vi "Initialize.vi"(8 "error in":errorcluster, 11 "Plugin in":refnum<class "Power Spectrum Density.lvclass">) -> (0 "error out":errorcluster, 3 "Plugin out":refnum<class "Power Spectrum Density.lvclass">)   [LabVIEW 2023, in "Power Spectrum Density.lvlib" / "Power Spectrum Density.lvclass"]
uses:
  Power Spectrum Density.lvclass
  C:/Program Files/National Instruments/LabVIEW 2023/vi.lib/FlexLogger/SDK/PluginSDK.lvlibp/PEFClasses/SDK/Plugin/Plugin.lvclass
  Power Spectrum Density Global.vi
  <vilib>/FlexLogger/SDK/PluginSDK.lvlibp/PEFClasses/SDK/Plugin/ParameterAccess/Write Single Channel.vi
  <vilib>/FlexLogger/SDK/PluginSDK.lvlibp/PEFClasses/SDK/Plugin/ParameterAccess/Write Enum.vi
  <vilib>/FlexLogger/SDK/PluginSDK.lvlibp/PEFClasses/SDK/Plugin/ParameterAccess/Write Boolean.vi
  <vilib>/FlexLogger/SDK/PluginSDK.lvlibp/PEFClasses/SDK/Plugin/ParameterAccess/Write I32.vi
  <vilib>/FlexLogger/SDK/PluginSDK.lvlibp/PEFClasses/SDK/Plugin/ParameterAccess/Write DBL.vi
  <vilib>/FlexLogger/SDK/PluginSDK.lvlibp/PEFClasses/SDK/Plugin/ParameterAccess/Write Command.vi
  <vilib>/FlexLogger/SDK/PluginSDK.lvlibp/PEFClasses/SDK/Plugin/Plugin.lvclass
  C:/Program Files/National Instruments/LabVIEW 2023/vi.lib/FlexLogger/SDK/PluginSDK.lvlibp/PEFClasses/SDK/Processing Element/Processing Element.lvclass
  C:/Users/Administrator/Documents/LabVIEW Projects/FlexLogger IO Plug-ins/Power Spectrum Density/Power Spectrum Density.lvclass
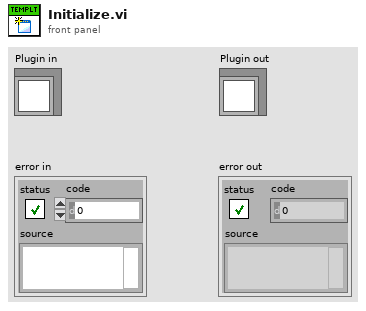
[diagram p1: front panel]
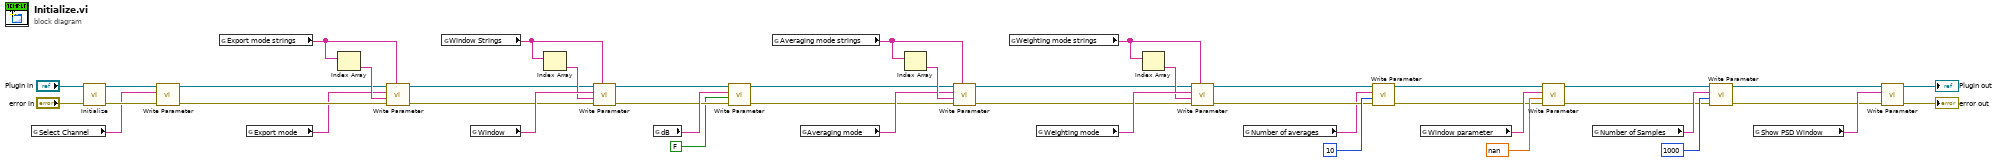
[diagram p0: block diagram]
diagram:
  n1 = global read "Power Spectrum Density Global.vi" "Select Channel"() -> (w38:string)
  n2 = call-parent "Initialize.vi"("error in (no error)"="error in", "Plugin in"="Plugin in") -> ("error out"=w39:errorcluster, "Plugin out"=w40:refnum<class "Power Spectrum Density.lvclass">)  [unwired: 8 in]
  n3 = call-poly <vilib>:"Write Parameter.vi"("error in (no error)"=w39, "Name (Unique Channel Identifier)"=w38, "Plugin in"=w40) -> ("error out"=w41:errorcluster, "Plugin out"=w42:refnum<class "Power Spectrum Density.lvclass">)  [unwired: 7 in]
  n4 = global read "Power Spectrum Density Global.vi" "Export mode strings"() -> (w37:string[])
  n5 = global read "Power Spectrum Density Global.vi" "Export mode"() -> (w36:string)
  n6 = Index Array(array=w37) -> (element=w43:string)  [unwired: 1 in]
  n7 = call-poly <vilib>:"Write Parameter.vi"("Possible Values"=w37, "error in (no error)"=w41, "Current Value"=w43, "Name"=w36, "Plugin in"=w42) -> ("error out"=w29:errorcluster, "Plugin out"=w30:refnum<class "Power Spectrum Density.lvclass">)  [unwired: 5 in]
  n8 = global read "Power Spectrum Density Global.vi" "Window Strings"() -> (w32:string[])
  n9 = global read "Power Spectrum Density Global.vi" "Window"() -> (w33:string)
  n10 = Index Array(array=w32) -> (element=w31:string)  [unwired: 1 in]
  n11 = call-poly <vilib>:"Write Parameter.vi"("Possible Values"=w32, "error in (no error)"=w29, "Current Value"=w31, "Name"=w33, "Plugin in"=w30) -> ("error out"=w26:errorcluster, "Plugin out"=w27:refnum<class "Power Spectrum Density.lvclass">)  [unwired: 5 in]
  n12 = global read "Power Spectrum Density Global.vi" "dB"() -> (w28:string)
  n13 = call-poly <vilib>:"Write Parameter.vi"("error in (no error)"=w26, "Value"=FALSE, "Name"=w28, "Plugin in"=w27) -> ("error out"=w17:errorcluster, "Plugin out"=w18:refnum<class "Power Spectrum Density.lvclass">)  [unwired: 6 in]
  n14 = global read "Power Spectrum Density Global.vi" "Averaging mode strings"() -> (w23:string[])
  n15 = global read "Power Spectrum Density Global.vi" "Averaging mode"() -> (w22:string)
  n16 = Index Array(array=w23) -> (element=w24:string)  [unwired: 1 in]
  n17 = call-poly <vilib>:"Write Parameter.vi"("Possible Values"=w23, "error in (no error)"=w17, "Current Value"=w24, "Name"=w22, "Plugin in"=w18) -> ("error out"=w15:errorcluster, "Plugin out"=w16:refnum<class "Power Spectrum Density.lvclass">)  [unwired: 5 in]
  n18 = global read "Power Spectrum Density Global.vi" "Weighting mode strings"() -> (w20:string[])
  n19 = global read "Power Spectrum Density Global.vi" "Weighting mode"() -> (w21:string)
  n20 = Index Array(array=w20) -> (element=w19:string)  [unwired: 1 in]
  n21 = call-poly <vilib>:"Write Parameter.vi"("Possible Values"=w20, "error in (no error)"=w15, "Current Value"=w19, "Name"=w21, "Plugin in"=w16) -> ("error out"=w13:errorcluster, "Plugin out"=w14:refnum<class "Power Spectrum Density.lvclass">)  [unwired: 5 in]
  n22 = global read "Power Spectrum Density Global.vi" "Number of averages"() -> (w12:string)
  n23 = call-poly <vilib>:"Write Parameter.vi"("error in (no error)"=w13, "Value"=10, "Name"=w12, "Plugin in"=w14) -> ("error out"=w8:errorcluster, "Plugin out"=w9:refnum<class "Power Spectrum Density.lvclass">)  [unwired: 6 in]
  n24 = global read "Power Spectrum Density Global.vi" "Window parameter"() -> (w11:string)
  n25 = call-poly <vilib>:"Write Parameter.vi"("error in (no error)"=w8, "Value"=nan, "Name"=w11, "Plugin in"=w9) -> ("error out"=w2:errorcluster, "Plugin out"=w4:refnum<class "Power Spectrum Density.lvclass">)  [unwired: 6 in]
  n26 = global read "Power Spectrum Density Global.vi" "Number of Samples"() -> (w6:string)
  n27 = call-poly <vilib>:"Write Parameter.vi"("error in (no error)"=w2, "Value"=1000, "Name"=w6, "Plugin in"=w4) -> ("error out"=w1:errorcluster, "Plugin out"=w3:refnum<class "Power Spectrum Density.lvclass">)  [unwired: 6 in]
  n28 = global read "Power Spectrum Density Global.vi" "Show PSD Window"() -> (w7:string)
  n29 = call-poly <vilib>:"Write Parameter.vi"("error in (no error)"=w1, "Name"=w7, "Plugin in"=w3) -> ("error out"=→"error out":errorcluster, "Plugin out"=→"Plugin out":refnum<class "Power Spectrum Density.lvclass">)  [unwired: 7 in]
